vi "3D创建.vi"() -> (0 "旋转臂":refnum<vi>, 1 "摆臂":refnum<vi>, 2 "底座":refnum<vi>)   [LabVIEW 2012]
uses:
  <vilib>/Utility/miscctls.llb/LV3DPointTypeDef.ctl
  <vilib>/picture/3D Picture Control/NI_3D Picture Control.lvlib
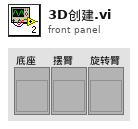
[diagram p1: front panel]
types:
  T1 = cluster{"Red":sgl, "Green":sgl, "Blue":sgl, "Alpha":sgl}
  T2 = typedef "LV3DPointTypeDef.ctl" = cluster{"X":sgl, "Y":sgl, "Z":sgl}
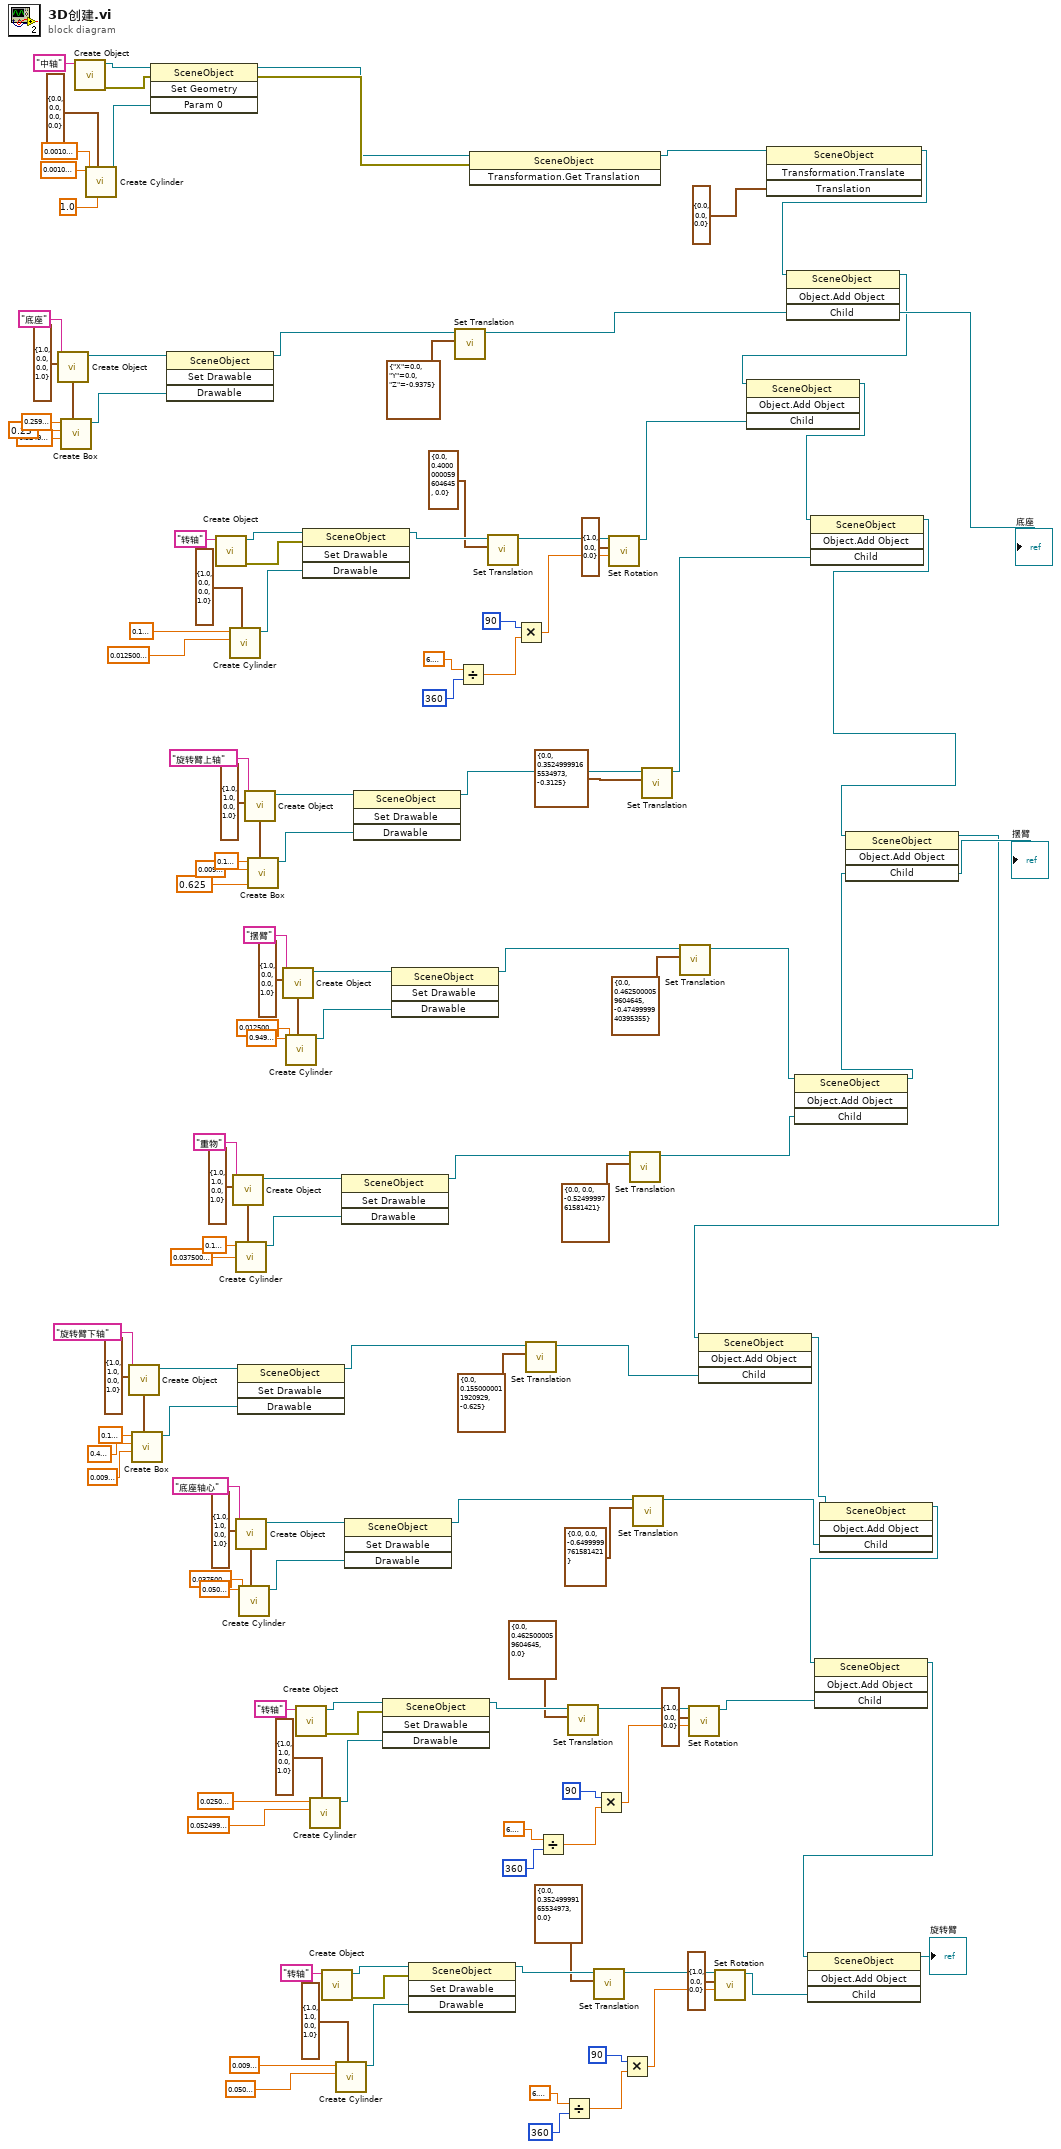
[diagram p0: block diagram]
diagram:
  n1 = call <vilib>:"Create Object.vi"("Name"="底座") -> ("Scene:New Object"=w75:refnum<vi>)  [unwired: 9 in, 1 out]
  n2 = call <vilib>:"Create Box.vi"("Color"=T1 {"Red"=1.0, "Green"=0.0, "Blue"=0.0, "Alpha"=1.0}, "Length Z"=sgl 0.525, "Length Y"=sgl 0.25, "Length X"=sgl 0.26) -> ("New Box Refnum"=w74:refnum<vi>)  [unwired: 6 in, 1 out]
  n3 = call <vilib>:"Create Object.vi"("Name"="中轴") -> ("error out"=w130:errorcluster, "Scene:New Object"=w123:refnum<vi>)  [unwired: 9 in]
  n4 = call <vilib>:"Create Cylinder.vi"("Detail"=sgl 1.0, "Color"=T1 {"Red"=0.0, "Green"=0.0, "Blue"=0.0, "Alpha"=0.0}, "Radius"=sgl 0.001, "Height"=sgl 0.001) -> ("New Cylinder Refnum"=w124:refnum<vi>)  [unwired: 6 in, 1 out]
  n5 = call <vilib>:"Create Object.vi"("Name"="旋转臂下轴") -> ("Scene:New Object"=w59:refnum<vi>)  [unwired: 9 in, 1 out]
  n6 = call <vilib>:"Create Box.vi"("Color"=T1 {"Red"=1.0, "Green"=1.0, "Blue"=0.0, "Alpha"=1.0}, "Length Z"=sgl 0.01, "Length Y"=sgl 0.4, "Length X"=sgl 0.1) -> ("New Box Refnum"=w58:refnum<vi>)  [unwired: 6 in, 1 out]
  n7 = invoke class="SceneObject" method="Set Geometry"(reference=w123, error in=w130, "Param 0"=w124) -> (reference out=w128:refnum<vi>, error out=w129:errorcluster)  [unwired: 1 in, 2 out]
  n8 = invoke class="SceneObject" method="Set Drawable"(reference=w75, "Drawable"=w74) -> (reference out=w73:refnum<vi>)  [unwired: 2 in, 3 out]
  n9 = call <vilib>:"Create Object.vi"("Name"="转轴") -> ("error out"=w100:errorcluster, "Scene:New Object"=w101:refnum<vi>)  [unwired: 9 in]
  n10 = call <vilib>:"Create Cylinder.vi"("Color"=T1 {"Red"=1.0, "Green"=0.0, "Blue"=0.0, "Alpha"=1.0}, "Radius"=sgl 0.0125, "Height"=sgl 0.1) -> ("New Cylinder Refnum"=w99:refnum<vi>)  [unwired: 7 in, 1 out]
  n11 = call <vilib>:"Create Object.vi"("Name"="重物") -> ("Scene:New Object"=w85:refnum<vi>)  [unwired: 9 in, 1 out]
  n12 = call <vilib>:"Create Cylinder.vi"("Color"=T1 {"Red"=1.0, "Green"=1.0, "Blue"=0.0, "Alpha"=1.0}, "Radius"=sgl 0.0375, "Height"=sgl 0.1) -> ("New Cylinder Refnum"=w84:refnum<vi>)  [unwired: 7 in, 1 out]
  n13 = call <vilib>:"Create Object.vi"("Name"="底座轴心") -> ("Scene:New Object"=w43:refnum<vi>)  [unwired: 9 in, 1 out]
  n14 = invoke class="SceneObject" method="Set Drawable"(reference=w59, "Drawable"=w58) -> (reference out=w57:refnum<vi>)  [unwired: 2 in, 3 out]
  n15 = call <vilib>:"Create Cylinder.vi"("Color"=T1 {"Red"=1.0, "Green"=1.0, "Blue"=0.0, "Alpha"=1.0}, "Radius"=sgl 0.0375, "Height"=sgl 0.05) -> ("New Cylinder Refnum"=w42:refnum<vi>)  [unwired: 7 in, 1 out]
  n16 = call <vilib>:"Create Object.vi"("Name"="旋转臂上轴") -> ("Scene:New Object"=w118:refnum<vi>)  [unwired: 9 in, 1 out]
  n17 = call <vilib>:"Create Box.vi"("Color"=T1 {"Red"=1.0, "Green"=1.0, "Blue"=0.0, "Alpha"=1.0}, "Length Z"=sgl 0.625, "Length Y"=sgl 0.01, "Length X"=sgl 0.1) -> ("New Box Refnum"=w117:refnum<vi>)  [unwired: 6 in, 1 out]
  n18 = call <vilib>:"Create Object.vi"("Name"="摆臂") -> ("Scene:New Object"=w110:refnum<vi>)  [unwired: 9 in, 1 out]
  n19 = call <vilib>:"Create Cylinder.vi"("Color"=T1 {"Red"=1.0, "Green"=0.0, "Blue"=0.0, "Alpha"=1.0}, "Radius"=sgl 0.0125, "Height"=sgl 0.95) -> ("New Cylinder Refnum"=w109:refnum<vi>)  [unwired: 7 in, 1 out]
  n20 = call <vilib>:"Create Object.vi"("Name"="转轴") -> ("error out"=w32:errorcluster, "Scene:New Object"=w33:refnum<vi>)  [unwired: 9 in]
  n21 = invoke class="SceneObject" method="Set Drawable"(reference=w101, error in=w100, "Drawable"=w99) -> (reference out=w98:refnum<vi>)  [unwired: 1 in, 3 out]
  n22 = call <vilib>:"Create Cylinder.vi"("Color"=T1 {"Red"=1.0, "Green"=1.0, "Blue"=0.0, "Alpha"=1.0}, "Radius"=sgl 0.0525, "Height"=sgl 0.025) -> ("New Cylinder Refnum"=w31:refnum<vi>)  [unwired: 7 in, 1 out]
  n23 = call <vilib>:"Create Object.vi"("Name"="转轴") -> ("error out"=w14:errorcluster, "Scene:New Object"=w15:refnum<vi>)  [unwired: 9 in]
  n24 = call <vilib>:"Create Cylinder.vi"("Color"=T1 {"Red"=1.0, "Green"=1.0, "Blue"=0.0, "Alpha"=1.0}, "Radius"=sgl 0.05, "Height"=sgl 0.01) -> ("New Cylinder Refnum"=w13:refnum<vi>)  [unwired: 7 in, 1 out]
  n25 = invoke class="SceneObject" method="Set Drawable"(reference=w85, "Drawable"=w84) -> (reference out=w83:refnum<vi>)  [unwired: 2 in, 3 out]
  n26 = invoke class="SceneObject" method="Set Drawable"(reference=w43, "Drawable"=w42) -> (reference out=w41:refnum<vi>)  [unwired: 2 in, 3 out]
  n27 = invoke class="SceneObject" method="Set Drawable"(reference=w118, "Drawable"=w117) -> (reference out=w116:refnum<vi>)  [unwired: 2 in, 3 out]
  n28 = invoke class="SceneObject" method="Set Drawable"(reference=w33, error in=w32, "Drawable"=w31) -> (reference out=w30:refnum<vi>)  [unwired: 1 in, 3 out]
  n29 = invoke class="SceneObject" method="Set Drawable"(reference=w110, "Drawable"=w109) -> (reference out=w108:refnum<vi>)  [unwired: 2 in, 3 out]
  n30 = invoke class="SceneObject" method="Set Drawable"(reference=w15, error in=w14, "Drawable"=w13) -> (reference out=w12:refnum<vi>)  [unwired: 1 in, 3 out]
  n31 = call <vilib>:"Set Translation.vi"("Translation"=cluster{"X":sgl, "Y":sgl, "Z":sgl} {"X"=0.0, "Y"=0.0, "Z"=-0.9375} ("Translation 2"), "Scene Object"=w73) -> ("Translated Object"=w71:refnum<vi>)  [unwired: 8 in, 1 out]
  n32 = Divide(x=6.283185307179586, y=360) -> (x/y=w92:dbl)
  n33 = invoke class="SceneObject" method="Transformation.Get Translation"(reference=w128, error in=w129) -> (reference out=w132:refnum<vi>)  [unwired: 1 in, 2 out]
  n34 = call <vilib>:"Set Translation.vi"("Translation"=cluster{"X":sgl, "Y":sgl, "Z":sgl} {"X"=0.0, "Y"=0.4, "Z"=0.0}, "Scene Object"=w98) -> ("Translated Object"=w96:refnum<vi>)  [unwired: 8 in, 1 out]
  n35 = Multiply(x=90, y=w92) -> (x*y=w90:dbl)
  n36 = call <vilib>:"Set Translation.vi"("Translation"=cluster{"X":sgl, "Y":sgl, "Z":sgl} {"X"=0.0, "Y"=0.155, "Z"=-0.625} ("Translation 2"), "Scene Object"=w57) -> ("Translated Object"=w52:refnum<vi>)  [unwired: 8 in, 1 out]
  n37 = Divide(x=6.283185307179586, y=360) -> (x/y=w24:dbl)
  n38 = Divide(x=6.283185307179586, y=360) -> (x/y=w6:dbl)
  n39 = call <vilib>:"Set Translation.vi"("Translation"=cluster{"X":sgl, "Y":sgl, "Z":sgl} {"X"=0.0, "Y"=0.4625, "Z"=0.0}, "Scene Object"=w30) -> ("Translated Object"=w28:refnum<vi>)  [unwired: 8 in, 1 out]
  n40 = call <vilib>:"Set Translation.vi"("Translation"=cluster{"X":sgl, "Y":sgl, "Z":sgl} {"X"=0.0, "Y"=0.3525, "Z"=0.0}, "Scene Object"=w12) -> ("Translated Object"=w10:refnum<vi>)  [unwired: 8 in, 1 out]
  n41 = Multiply(x=90, y=w24) -> (x*y=w22:dbl)
  n42 = call <vilib>:"Set Rotation.vi"("Angle"=w90, "Axis"=cluster{"X":sgl, "Y":sgl, "Z":sgl} {"X"=1.0, "Y"=0.0, "Z"=0.0}, "Scene Object"=w96) -> ("Rotated Scene Object"=w63:refnum<vi>)  [unwired: 7 in, 1 out]
  n43 = Multiply(x=90, y=w6) -> (x*y=w4:dbl)
  n44 = call <vilib>:"Set Translation.vi"("Translation"=cluster{"X":sgl, "Y":sgl, "Z":sgl} {"X"=0.0, "Y"=0.0, "Z"=-0.525} ("Translation 2"), "Scene Object"=w83) -> ("Translated Object"=w81:refnum<vi>)  [unwired: 8 in, 1 out]
  n45 = call <vilib>:"Set Translation.vi"("Translation"=cluster{"X":sgl, "Y":sgl, "Z":sgl} {"X"=0.0, "Y"=0.0, "Z"=-0.65} ("Translation 2"), "Scene Object"=w41) -> ("Translated Object"=w39:refnum<vi>)  [unwired: 8 in, 1 out]
  n46 = call <vilib>:"Set Translation.vi"("Translation"=cluster{"X":sgl, "Y":sgl, "Z":sgl} {"X"=0.0, "Y"=0.3525, "Z"=-0.3125}, "Scene Object"=w116) -> ("Translated Object"=w78:refnum<vi>)  [unwired: 8 in, 1 out]
  n47 = call <vilib>:"Set Translation.vi"("Translation"=cluster{"X":sgl, "Y":sgl, "Z":sgl} {"X"=0.0, "Y"=0.4625, "Z"=-0.475} ("Translation 2"), "Scene Object"=w108) -> ("Translated Object"=w80:refnum<vi>)  [unwired: 8 in, 1 out]
  n48 = call <vilib>:"Set Rotation.vi"("Angle"=w22, "Axis"=cluster{"X":sgl, "Y":sgl, "Z":sgl} {"X"=1.0, "Y"=0.0, "Z"=0.0}, "Scene Object"=w28) -> ("Rotated Scene Object"=w20:refnum<vi>)  [unwired: 7 in, 1 out]
  n49 = call <vilib>:"Set Rotation.vi"("Angle"=w4, "Axis"=cluster{"X":sgl, "Y":sgl, "Z":sgl} {"X"=1.0, "Y"=0.0, "Z"=0.0}, "Scene Object"=w10) -> ("Rotated Scene Object"=w3:refnum<vi>)  [unwired: 7 in, 1 out]
  n50 = invoke class="SceneObject" method="Transformation.Translate"(reference=w132, "Translation"=T2 {"X"=0.0, "Y"=0.0, "Z"=0.0} ("变换")) -> (reference out=w67:refnum<vi>)  [unwired: 2 in, 3 out]
  n51 = invoke class="SceneObject" method="Object.Add Object"(reference=w67, "Child"=w71) -> (reference out=w64:refnum<vi>, "Child"=→"底座":refnum<vi>)  [unwired: 2 in, 2 out]
  n52 = invoke class="SceneObject" method="Object.Add Object"(reference=w64, "Child"=w63) -> (reference out=w62:refnum<vi>)  [unwired: 2 in, 3 out]
  n53 = invoke class="SceneObject" method="Object.Add Object"(reference=w80, "Child"=w81) -> (reference out=w79:refnum<vi>)  [unwired: 2 in, 3 out]
  n54 = invoke class="SceneObject" method="Object.Add Object"(reference=w62, "Child"=w78) -> (reference out=w66:refnum<vi>)  [unwired: 2 in, 3 out]
  n55 = invoke class="SceneObject" method="Object.Add Object"(reference=w66, "Child"=w79) -> (reference out=w51:refnum<vi>, "Child"=→"摆臂":refnum<vi>)  [unwired: 2 in, 2 out]
  n56 = invoke class="SceneObject" method="Object.Add Object"(reference=w51, "Child"=w52) -> (reference out=w38:refnum<vi>)  [unwired: 2 in, 3 out]
  n57 = invoke class="SceneObject" method="Object.Add Object"(reference=w38, "Child"=w39) -> (reference out=w21:refnum<vi>)  [unwired: 2 in, 3 out]
  n58 = invoke class="SceneObject" method="Object.Add Object"(reference=w21, "Child"=w20) -> (reference out=w2:refnum<vi>)  [unwired: 2 in, 3 out]
  n59 = invoke class="SceneObject" method="Object.Add Object"(reference=w2, "Child"=w3) -> (reference out=→"旋转臂":refnum<vi>)  [unwired: 2 in, 3 out]
